vi "DereferencingPointerTo2DArrayOfIntegers.vi"(8 "error in (no error)":errorcluster, 9 "Cols":i32, 10 "Rows":i32, 11 "Address (Pointer)":i64) -> (0 "error out":errorcluster, 3 "Value":i32[][](array[numeric]))   [LabVIEW 2009, in "LabVIEWWrapper_PassingDataSampleDLL.lvlib"]
uses:
  LabVIEWWrapper_PassingDataSampleDLL.lvlib
  <vilib>/Utility/importsl/GetValueByPointer/GetValueByPointer.xnode
  <vilib>/Utility/importsl/GetValueByPointer/datatype.ctl
  Program Files (x86)/National Instruments/LabVIEW 2009/resource/lvimptsl.dll
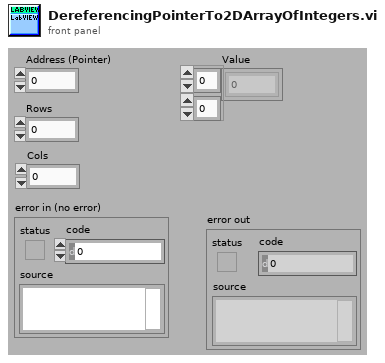
[diagram p1: front panel]
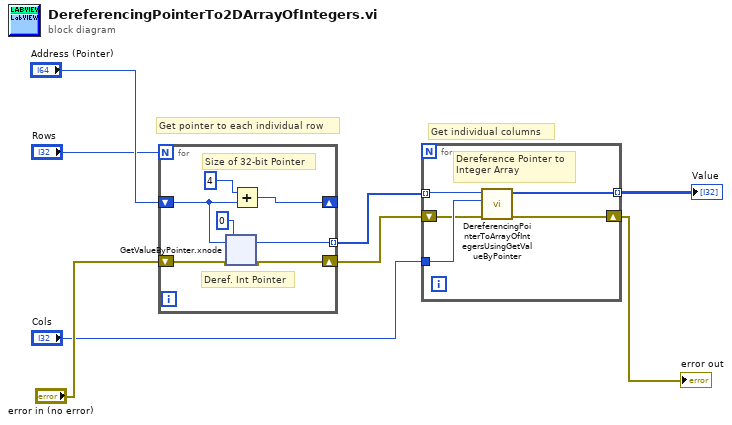
[diagram p0: block diagram]
diagram:
  # "Get individual columns"
  # "Get pointer to each individual row"
  n1 = for {
    N: "Rows" -> [_]
    shift-right: [w14] -> _
    shift-left: "Address (Pointer)" -> [w13]
    shift-right: [w10] -> w3
    shift-left: "error in (no error)" -> [w11]
    tunnel: [w9] -> w5 mode=indexing
    # "Deref. Int Pointer"
    # "Size of 32-bit Pointer"
    n2 = xnode "GetValueByPointer.xnode"("Pointer"=w13, "InputType"=i64 0, "ErrorIn"=w11) -> ("Output"=w9:i64, "ErrorOut"=w10:errorcluster)  [unwired: 1 in]
    n3 = Add(x=i64 4, y=w13) -> (x+y=w14:i64)
  }
  n4 = for {
    tunnel: w5 -> [w28] mode=indexing
    tunnel: "Cols" -> [w27]
    shift-right: [w25] -> w1
    shift-left: w3 -> [w26]
    tunnel: [w24] -> w2 mode=indexing
    # "Dereference Pointer to\nInteger Array"
    n5 = call "DereferencingPointerToArrayOfIntegersUsingGetValueByPointer.vi"("error in (no error)"=w26, "Length"=w27, "Address (Pointer)"=w28) -> ("error out"=w25:errorcluster, "Value"=w24:i32[])  [unwired: 7 in]
  }
  "error out" <- w1
  "Value" <- w2
